vi "main.vi"() -> ()   [LabVIEW 2023] (continued)
1FFFFFFF   00000004    8        00\t00\tFF\tFF\tFF\tFF\tFF\tFF\r\n      3246  18F121F0   00000004    8        09\t33\t00\t00\tFF\tFF\tB0\t01\r\n      3245  18F106A7   00000004    8        00\tF7\tFF\tFF\tFF\tFF\tFF\tB1\r\n      3245  0CF104A7   00000004    8        F0\t60\t22\tFC\tFF\tFF\tFF\t58\r\n      3244  0CF103A7   00000004    8        17\t1F\t08\t60\tB1\t1F\t08\t58\r\n      3244  0CF102A7   00000004    8        30\t75\tE0\t2E\t80\tFF\tFF\tFD\r\n      3243  0C3C4D4A   00000004    8        BE\tFF\tFF\t7F\t18\tFF\tFF\t58\r\n      3272  1FFFFFFF   00000004    8        00\t00\tFF\tFF\tFF\tFF\tFF\tFF\r\n      3263  0CF102A7   00000004    8        30\t75\tE0\t2E\t80\tFF\tFF\tFD\r\n      3263  0CF101A7   00000004    8        68\t00\t97\tCC\t00\t19\t39\tBD\r\n      3262  1FFFFFFF   00000004    8        00\t00\tFF\tFF\tFF\tFF\tFF\tFF\r\n      3252  1FFFFFFF   00000004    8        00\t00\tFF\tFF\tFF\tFF\tFF\tFF\r\n      3247  1FFFFFFF   00000004    8        00\t00\tFF\tFF\tFF\tFF\tFF\tFF\r\n      3246  18F121F0   00000004    8        09\t33\t00\t00\tFF\tFF\tB0\t01\r\n      3245  18F106A7   00000004    8        00\tF7\tFF\tFF\tFF\tFF\tFF\tB1\r\n      3245  0CF104A7   00000004    8        F0\t60\t22\tFC\tFF\tFF\tFF\t58\r\n      3244  0CF103A7   00000004    8        17\t1F\t08\t60\tB1\t1F\t08\t58\r\n      3244  0CF102A7   00000004    8        30\t75\tE0\t2E\t80\tFF\tFF\tFD\r\n      3282  1FFFFFFF   00000004    8        00\t00\tFF\tFF\tFF\tFF\tFF\tFF\r\n      3272  1FFFFFFF   00000004    8        00\t00\tFF\tFF\tFF\tFF\tFF\tFF\r\n      3263  0CF102A7   00000004    8        30\t75\tE0\t2E\t80\tFF\tFF\tFD\r\n      3263  0CF101A7   00000004    8        68\t00\t97\tCC\t00\t19\t39\tBD\r\n      3262  1FFFFFFF   00000004    8        00\t00\tFF\tFF\tFF\tFF\tFF\tFF\r\n      3252  1FFFFFFF   00000004    8        00\t00\tFF\tFF\tFF\tFF\tFF\tFF\r\n      3247  1FFFFFFF   00000004    8        00\t00\tFF\tFF\tFF\tFF\tFF\tFF\r\n      3246  18F121F0   00000004    8        09\t33\t00\t00\tFF\tFF\tB0\t01\r\n      3245  18F106A7   00000004    8        00\tF7\tFF\tFF\tFF\tFF\tFF\tB1\r\n      3245  0CF104A7   00000004    8        F0\t60\t22\tFC\tFF\tFF\tFF\t58\r\n      3244  0CF103A7   00000004    8        17\t1F\t08\t60\tB1\t1F\t08\t58\r\n      3283  0CF101A7   00000004    8        68\t00\t97\tCC\t00\t19\t39\tBE\r\n      3282  1FFFFFFF   00000004    8        00\t00\tFF\tFF\tFF\tFF\tFF\tFF\r\n      3272  1FFFFFFF   00000004    8        00\t00\tFF\tFF\tFF\tFF\tFF\tFF\r\n      3263  0CF102A7   00000004    8        30\t75\tE0\t2E\t80\tFF\tFF\tFD\r\n      3263  0CF101A7   00000004    8        68\t00\t97\tCC\t00\t19\t39\tBD\r\n      3262  1FFFFFFF   00000004    8        00\t00\tFF\tFF\tFF\tFF\tFF\tFF\r\n      3252  1FFFFFFF   00000004    8        00\t00\tFF\tFF\tFF\tFF\tFF\tFF\r\n      3247  1FFFFFFF   00000004    8        00\t00\tFF\tFF\tFF\tFF\tFF\tFF\r\n      3246  18F121F0   00000004    8        09\t33\t00\t00\tFF\tFF\tB0\t01\r\n      3245  18F106A7   00000004    8        00\tF7\tFF\tFF\tFF\tFF\tFF\tB1\r\n      3245  0CF104A7   00000004    8        F0\t60\t22\tFC\tFF\tFF\tFF\t58\r\n      3283  0CF102A7   00000004    8        30\t75\tE0\t2E\t80\tFF\tFF\tFD\r\n      3283  0CF101A7   00000004    8        68\t00\t97\tCC\t00\t19\t39\tBE\r\n      3282  1FFFFFFF   00000004    8        00\t00\tFF\tFF\tFF\tFF\tFF\tFF\r\n      3272  1FFFFFFF   00000004    8        00\t00\tFF\tFF\tFF\tFF\tFF\tFF\r\n      3263  0CF102A7   00000004    8        30\t75\tE0\t2E\t80\tFF\tFF\tFD\r\n      3263  0CF101A7   00000004    8        68\t00\t97\tCC\t00\t19\t39\tBD\r\n      3262  1FFFFFFF   00000004    8        00\t00\tFF\tFF\tFF\tFF\tFF\tFF\r\n      3252  1FFFFFFF   00000004    8        00\t00\tFF\tFF\tFF\tFF\tFF\tFF\r\n      3247  1FFFFFFF   00000004    8        00\t00\tFF\tFF\tFF\tFF\tFF\tFF\r\n      3246  18F121F0   00000004    8        09\t33\t00\t00\tFF\tFF\tB0\t01\r\n      3245  18F106A7   00000004    8        00\tF7\tFF\tFF\tFF\tFF\tFF\tB1\r\n      3292  1FFFFFFF   00000004    8        00\t00\tFF\tFF\tFF\tFF\tFF\tFF\r\n      3283  0CF102A7   00000004    8        30\t75\tE0\t2E\t80\tFF\tFF\tFD\r\n      3283  0CF101A7   00000004    8        68\t00\t97\tCC\t00\t19\t39\tBE\r\n      3282  1FFFFFFF   00000004    8        00\t00\tFF\tFF\tFF\tFF\tFF\tFF\r\n      3272  1FFFFFFF   00000004    8        00\t00\tFF\tFF\tFF\tFF\tFF\tFF\r\n      3263  0CF102A7   00000004    8        30\t75\tE0\t2E\t80\tFF\tFF\tFD\r\n      3263  0CF101A7   00000004    8        68\t00\t97\tCC\t00\t19\t39\tBD\r\n      3262  1FFFFFFF   00000004    8        00\t00\tFF\tFF\tFF\tFF\tFF\tFF\r\n      3252  1FFFFFFF   00000004    8        00\t00\tFF\tFF\tFF\tFF\tFF\tFF\r\n      3247  1FFFFFFF   00000004    8        00\t00\tFF\tFF\tFF\tFF\tFF\tFF\r\n      3246  18F121F0   00000004    8        09\t33\t00\t00\tFF\tFF\tB0\t01\r\n      3293  18F106A7   00000004    8        00\tF7\tFF\tFF\tFF\tFF\tFF\tB2\r\n      3292  1FFFFFFF   00000004    8        00\t00\tFF\tFF\tFF\tFF\tFF\tFF\r\n      3283  0CF102A7   00000004    8        30\t75\tE0\t2E\t80\tFF\tFF\tFD\r\n      3283  0CF101A7   00000004    8        68\t00\t97\tCC\t00\t19\t39\tBE\r\n      3282  1FFFFFFF   00000004    8        00\t00\tFF\tFF\tFF\tFF\tFF\tFF\r\n      3272  1FFFFFFF   00000004    8        00\t00\tFF\tFF\tFF\tFF\tFF\tFF\r\n      3263  0CF102A7   00000004    8        30\t75\tE0\t2E\t80\tFF\tFF\tFD\r\n      3263  0CF101A7   00000004    8        68\t00\t97\tCC\t00\t19\t39\tBD\r\n      3262  1FFFFFFF   00000004    8        00\t00\tFF\tFF\tFF\tFF\tFF\tFF\r\n      3252  1FFFFFFF   00000004    8        00\t00\tFF\tFF\tFF\tFF\tFF\tFF\r\n      3247  1FFFFFFF   00000004    8        00\t00\tFF\tFF\tFF\tFF\tFF\tFF\r\n      3302  1FFFFFFF   00000004    8        00\t00\tFF\tFF\tFF\tFF\tFF\tFF\r\n      3293  18F106A7   00000004    8        00\tF7\tFF\tFF\tFF\tFF\tFF\tB2\r\n      3292  1FFFFFFF   00000004    8        00\t00\tFF\tFF\tFF\tFF\tFF\tFF\r\n      3283  0CF102A7   00000004    8        30\t75\tE0\t2E\t80\tFF\tFF\tFD\r\n      3283  0CF101A7   00000004    8        68\t00\t97\tCC\t00\t19\t39\tBE\r\n      3282  1FFFFFFF   00000004    8        00\t00\tFF\tFF\tFF\tFF\tFF\tFF\r\n      3272  1FFFFFFF   00000004    8        00\t00\tFF\tFF\tFF\tFF\tFF\tFF\r\n      3263  0CF102A7   00000004    8        30\t75\tE0\t2E\t80\tFF\tFF\tFD\r\n      3263  0CF101A7   00000004    8        68\t00\t97\tCC\t00\t19\t39\tBD\r\n      3262  1FFFFFFF   00000004    8        00\t00\tFF\tFF\tFF\tFF\tFF\tFF\r\n      3252  1FFFFFFF   00000004    8        00\t00\tFF\tFF\tFF\tFF\tFF\tFF\r\n      3303  0CF101A7   00000004    8        68\t00\t97\tCC\t00\t19\t39\tBF\r\n      3302  1FFFFFFF   00000004    8        00\t00\tFF\tFF\tFF\tFF\tFF\tFF\r\n      3293  18F106A7   00000004    8        00\tF7\tFF\tFF\tFF\tFF\tFF\tB2\r\n      3292  1FFFFFFF   00000004    8        00\t00\tFF\tFF\tFF\tFF\tFF\tFF\r\n      3283  0CF102A7   00000004    8        30\t75\tE0\t2E\t80\tFF\tFF\tFD\r\n      3283  0CF101A7   00000004    8        68\t00\t97\tCC\t00\t19\t39\tBE\r\n      3282  1FFFFFFF   00000004    8        00\t00\tFF\tFF\tFF\tFF\tFF\tFF\r\n      3272  1FFFFFFF   00000004    8        00\t00\tFF\tFF\tFF\tFF\tFF\tFF\r\n      3263  0CF102A7   00000004    8        30\t75\tE0\t2E\t80\tFF\tFF\tFD\r\n      3263  0CF101A7   00000004    8        68\t00\t97\tCC\t00\t19\t39\tBD\r\n      3262  1FFFFFFF   00000004    8        00\t00\tFF\tFF\tFF\tFF\tFF\tFF\r\n      3303  0CF102A7   00000004    8        30\t75\tE0\t2E\t80\tFF\tFF\tFD\r\n      3303  0CF101A7   00000004    8        68\t00\t97\tCC\t00\t19\t39\tBF\r\n      3302  1FFFFFFF   00000004    8        00\t00\tFF\tFF\tFF\tFF\tFF\tFF\r\n      3293  18F106A7   00000004    8        00\tF7\tFF\tFF\tFF\tFF\tFF\tB2\r\n      3292  1FFFFFFF   00000004    8        00\t00\tFF\tFF\tFF\tFF\tFF\tFF\r\n      3283  0CF102A7   00000004    8        30\t75\tE0\t2E\t80\tFF\tFF\tFD\r\n      3283  0CF101A7   00000004    8        68\t00\t97\tCC\t00\t19\t39\tBE\r\n      3282  1FFFFFFF   00000004    8        00\t00\tFF\tFF\tFF\tFF\tFF\tFF\r\n      3272  1FFFFFFF   00000004    8        00\t00\tFF\tFF\tFF\tFF\tFF\tFF\r\n      3263  0CF102A7   00000004    8        30\t75\tE0\t2E\t80\tFF\tFF\tFD\r\n      3263  0CF101A7   00000004    8        68\t00\t97\tCC\t00\t19\t39\tBD\r\n      3312  1FFFFFFF   00000004    8        00\t20\tFF\tFF\tFF\tFF\tFF\tFF\r\n      3303  0CF102A7   00000004    8        30\t75\tE0\t2E\t80\tFF\tFF\tFD\r\n      3303  0CF101A7   00000004    8        68\t00\t97\tCC\t00\t19\t39\tBF\r\n      3302  1FFFFFFF   00000004    8        00\t00\tFF\tFF\tFF\tFF\tFF\tFF\r\n      3293  18F106A7   00000004    8        00\tF7\tFF\tFF\tFF\tFF\tFF\tB2\r\n      3292  1FFFFFFF   00000004    8        00\t00\tFF\tFF\tFF\tFF\tFF\tFF\r\n      3283  0CF102A7   00000004    8        30\t75\tE0\t2E\t80\tFF\tFF\tFD\r\n      3283  0CF101A7   00000004    8        68\t00\t97\tCC\t00\t19\t39\tBE\r\n      3282  1FFFFFFF   00000004    8        00\t00\tFF\tFF\tFF\tFF\tFF\tFF\r\n      3272  1FFFFFFF   00000004    8        00\t00\tFF\tFF\tFF\tFF\tFF\tFF\r\n      3263  0CF102A7   00000004    8        30\t75\tE0\t2E\t80\tFF\tFF\tFD\r\n      3322  1FFFFFFF   00000004    8        00\t00\tFF\tFF\tFF\tFF\tFF\tFF\r\n      3312  1FFFFFFF   00000004    8        00\t20\tFF\tFF\tFF\tFF\tFF\tFF\r\n      3303  0CF102A7   00000004    8        30\t75\tE0\t2E\t80\tFF\tFF\tFD\r\n      3303  0CF101A7   00000004    8        68\t00\t97\tCC\t00\t19\t39\tBF\r\n      3302  1FFFFFFF   00000004    8        00\t00\tFF\tFF\tFF\tFF\tFF\tFF\r\n      3293  18F106A7   00000004    8        00\tF7\tFF\tFF\tFF\tFF\tFF\tB2\r\n      3292  1FFFFFFF   00000004    8        00\t00\tFF\tFF\tFF\tFF\tFF\tFF\r\n      3283  0CF102A7   00000004    8        30\t75\tE0\t2E\t80\tFF\tFF\tFD\r\n      3283  0CF101A7   00000004    8        68\t00\t97\tCC\t00\t19\t39\tBE\r\n      3282  1FFFFFFF   00000004    8        00\t00\tFF\tFF\tFF\tFF\tFF\tFF\r\n      3272  1FFFFFFF   00000004    8        00\t00\tFF\tFF\tFF\tFF\tFF\tFF\r\n      3323  0CF101A7   00000004    8        68\t00\t97\tCC\t00\t19\t39\tC0\r\n      3322  1FFFFFFF   00000004    8        00\t00\tFF\tFF\tFF\tFF\tFF\tFF\r\n      3312  1FFFFFFF   00000004    8        00\t20\tFF\tFF\tFF\tFF\tFF\tFF\r\n      3303  0CF102A7   00000004    8        30\t75\tE0\t2E\t80\tFF\tFF\tFD\r\n      3303  0CF101A7   00000004    8        68\t00\t97\tCC\t00\t19\t39\tBF\r\n      3302  1FFFFFFF   00000004    8        00\t00\tFF\tFF\tFF\tFF\tFF\tFF\r\n      3293  18F106A7   00000004    8        00\tF7\tFF\tFF\tFF\tFF\tFF\tB2\r\n      3292  1FFFFFFF   00000004    8        00\t00\tFF\tFF\tFF\tFF\tFF\tFF\r\n      3283  0CF102A7   00000004    8        30\t75\tE0\t2E\t80\tFF\tFF\tFD\r\n      3283  0CF101A7   00000004    8        68\t00\t97\tCC\t00\t19\t39\tBE\r\n      3282  1FFFFFFF   00000004    8        00\t00\tFF\tFF\tFF\tFF\tFF\tFF\r\n      3323  0CF102A7   00000004    8        30\t75\tE0\t2E\t80\tFF\tFF\tFD\r\n      3323  0CF101A7   00000004    8        68\t00\t97\tCC\t00\t19\t39\tC0\r\n      3322  1FFFFFFF   00000004    8        00\t00\tFF\tFF\tFF\tFF\tFF\tFF\r\n      3312  1FFFFFFF   00000004    8        00\t20\tFF\tFF\tFF\tFF\tFF\tFF\r\n      3303  0CF102A7   00000004    8        30\t75\tE0\t2E\t80\tFF\tFF\tFD\r\n      3303  0CF101A7   00000004    8        68\t00\t97\tCC\t00\t19\t39\tBF\r\n      3302  1FFFFFFF   00000004    8        00\t00\tFF\tFF\tFF\tFF\tFF\tFF\r\n      3293  18F106A7   00000004    8        00\tF7\tFF\tFF\tFF\tFF\tFF\tB2\r\n      3292  1FFFFFFF   00000004    8        00\t00\tFF\tFF\tFF\tFF\tFF\tFF\r\n      3283  0CF102A7   00000004    8        30\t75\tE0\t2E\t80\tFF\tFF\tFD\r\n      3283  0CF101A7   00000004    8        68\t00\t97\tCC\t00\t19\t39\tBE\r\n      3332  1FFFFFFF   00000004    8        00\t00\tFF\tFF\tFF\tFF\tFF\tFF\r\n      3323  0CF102A7   00000004    8        30\t75\tE0\t2E\t80\tFF\tFF\tFD\r\n      3323  0CF101A7   00000004    8        68\t00\t97\tCC\t00\t19\t39\tC0\r\n      3322  1FFFFFFF   00000004    8        00\t00\tFF\tFF\tFF\tFF\tFF\tFF\r\n      3312  1FFFFFFF   00000004    8        00\t20\tFF\tFF\tFF\tFF\tFF\tFF\r\n      3303  0CF102A7   00000004    8        30\t75\tE0\t2E\t80\tFF\tFF\tFD\r\n      3303  0CF101A7   00000004    8        68\t00\t97\tCC\t00\t19\t39\tBF\r\n      3302  1FFFFFFF   00000004    8        00\t00\tFF\tFF\tFF\tFF\tFF\tFF\r\n      3293  18F106A7   00000004    8        00\tF7\tFF\tFF\tFF\tFF\tFF\tB2\r\n      3292  1FFFFFFF   00000004    8        00\t00\tFF\tFF\tFF\tFF\tFF\tFF\r\n      3283  0CF102A7   00000004    8        30\t75\tE0\t2E\t80\tFF\tFF\tFD\r\n      3341  18F11FF0   00000004    8        FF\t3F\t90\t68\t88\t1B\t10\t9C\r\n      3332  1FFFFFFF   00000004    8        00\t00\tFF\tFF\tFF\tFF\tFF\tFF\r\n      3323  0CF102A7   00000004    8        30\t75\tE0\t2E\t80\tFF\tFF\tFD\r\n      3323  0CF101A7   00000004    8        68\t00\t97\tCC\t00\t19\t39\tC0\r\n      3322  1FFFFFFF   00000004    8        00\t00\tFF\tFF\tFF\tFF\tFF\tFF\r\n      3312  1FFFFFFF   00000004    8        00\t20\tFF\tFF\tFF\tFF\tFF\tFF\r\n      3303  0CF102A7   00000004    8        30\t75\tE0\t2E\t80\tFF\tFF\tFD\r\n      3303  0CF101A7   00000004    8        68\t00\t97\tCC\t00\t19\t39\tBF\r\n      3302  1FFFFFFF   00000004    8        00\t00\tFF\tFF\tFF\tFF\tFF\tFF\r\n      3293  18F106A7   00000004    8        00\tF7\tFF\tFF\tFF\tFF\tFF\tB2\r\n      3292  1FFFFFFF   00000004    8        00\t00\tFF\tFF\tFF\tFF\tFF\tFF\r\n      3342  18F120F0   00000004    8        2B\t75\t60\tB1\tB0\t01\tFF\tFF\r\n      3341  18F11FF0   00000004    8        FF\t3F\t90\t68\t88\t1B\t10\t9C\r\n      3332  1FFFFFFF   00000004    8        00\t00\tFF\tFF\tFF\tFF\tFF\tFF\r\n      3323  0CF102A7   00000004    8        30\t75\tE0\t2E\t80\tFF\tFF\tFD\r\n      3323  0CF101A7   00000004    8        68\t00\t97\tCC\t00\t19\t39\tC0\r\n      3322  1FFFFFFF   00000004    8        00\t00\tFF\tFF\tFF\tFF\tFF\tFF\r\n      3312  1FFFFFFF   00000004    8        00\t20\tFF\tFF\tFF\tFF\tFF\tFF\r\n      3303  0CF102A7   00000004    8        30\t75\tE0\t2E\t80\tFF\tFF\tFD\r\n      3303  0CF101A7   00000004    8        68\t00\t97\tCC\t00\t19\t39\tBF\r\n      3302  1FFFFFFF   00000004    8        00\t00\tFF\tFF\tFF\tFF\tFF\tFF\r\n      3293  18F106A7   00000004    8        00\tF7\tFF\tFF\tFF\tFF\tFF\tB2\r\n      3343  0CF101A7   00000004    8        68\t00\t97\tCC\t00\t19\t39\tC1\r\n      3342  18F120F0   00000004    8        2B\t75\t60\tB1\tB0\t01\tFF\tFF\r\n      3341  18F11FF0   00000004    8        FF\t3F\t90\t68\t88\t1B\t10\t9C\r\n      3332  1FFFFFFF   00000004    8        00\t00\tFF\tFF\tFF\tFF\tFF\tFF\r\n      3323  0CF102A7   00000004    8        30\t75\tE0\t2E\t80\tFF\tFF\tFD\r\n      3323  0CF101A7   00000004    8        68\t00\t97\tCC\t00\t19\t39\tC0\r\n      3322  1FFFFFFF   00000004    8        00\t00\tFF\tFF\tFF\tFF\tFF\tFF\r\n      3312  1FFFFFFF   00000004    8        00\t20\tFF\tFF\tFF\tFF\tFF\tFF\r\n      3303  0CF102A7   00000004    8        30\t75\tE0\t2E\t80\tFF\tFF\tFD\r\n      3303  0CF101A7   00000004    8        68\t00\t97\tCC\t00\t19\t39\tBF\r\n      3302  1FFFFFFF   00000004    8        00\t00\tFF\tFF\tFF\tFF\tFF\tFF\r\n      3343  0C3C4D4A   00000004    8        BE\tFF\tFF\t7F\t18\tFF\tFF\t59\r\n      3343  0CF101A7   00000004    8        68\t00\t97\tCC\t00\t19\t39\tC1\r\n      3342  18F120F0   00000004    8        2B\t75\t60\tB1\tB0\t01\tFF\tFF\r\n      3341  18F11FF0   00000004    8        FF\t3F\t90\t68\t88\t1B\t10\t9C\r\n      3332  1FFFFFFF   00000004    8        00\t00\tFF\tFF\tFF\tFF\tFF\tFF\r\n      3323  0CF102A7   00000004    8        30\t75\tE0\t2E\t80\tFF\tFF\tFD\r\n      3323  0CF101A7   00000004    8        68\t00\t97\tCC\t00\t19\t39\tC0\r\n      3322  1FFFFFFF   00000004    8        00\t00\tFF\tFF\tFF\tFF\tFF\tFF\r\n      3312  1FFFFFFF   00000004    8        00\t20\tFF\tFF\tFF\tFF\tFF\tFF\r\n      3303  0CF102A7   00000004    8        30\t75\tE0\t2E\t80\tFF\tFF\tFD\r\n      3303  0CF101A7   00000004    8        68\t00\t97\tCC\t00\t19\t39\tBF\r\n      3344  0CF102A7   00000004    8        30\t75\tE0\t2E\t80\tFF\tFF\tFD\r\n      3343  0C3C4D4A   00000004    8        BE\tFF\tFF\t7F\t18\tFF\tFF\t59\r\n      3343  0CF101A7   00000004    8        68\t00\t97\tCC\t00\t19\t39\tC1\r\n      3342  18F120F0   00000004    8        2B\t75\t60\tB1\tB0\t01\tFF\tFF\r\n      3341  18F11FF0   00000004    8        FF\t3F\t90\t68\t88\t1B\t10\t9C\r\n      3332  1FFFFFFF   00000004    8        00\t00\tFF\tFF\tFF\tFF\tFF\tFF\r\n      3323  0CF102A7   00000004    8        30\t75\tE0\t2E\t80\tFF\tFF\tFD\r\n      3323  0CF101A7   00000004    8        68\t00\t97\tCC\t00\t19\t39\tC0\r\n      3322  1FFFFFFF   00000004    8        00\t00\tFF\tFF\tFF\tFF\tFF\tFF\r\n      3312  1FFFFFFF   00000004    8        00\t20\tFF\tFF\tFF\tFF\tFF\tFF\r\n      3303  0CF102A7   00000004    8        30\t75\tE0\t2E\t80\tFF\tFF\tFD\r\n      3344  0CF103A7   00000004    8        17\t1F\t08\t60\tB1\t1F\t08\t59\r\n      3344  0CF102A7   00000004    8        30\t75\tE0\t2E\t80\tFF\tFF\tFD\r\n      3343  0C3C4D4A   00000004    8        BE\tFF\tFF\t7F\t18\tFF\tFF\t59\r\n      3343  0CF101A7   00000004    8        68\t00\t97\tCC\t00\t19\t39\tC1\r\n      3342  18F120F0   00000004    8        2B\t75\t60\tB1\tB0\t01\tFF\tFF\r\n      3341  18F11FF0   00000004    8        FF\t3F\t90\t68\t88\t1B\t10\t9C\r\n      3332  1FFFFFFF   00000004    8        00\t00\tFF\tFF\tFF\tFF\tFF\tFF\r\n      3323  0CF102A7   00000004    8        30\t75\tE0\t2E\t80\tFF\tFF\tFD\r\n      3323  0CF101A7   00000004    8        68\t00\t97\tCC\t00\t19\t39\tC0\r\n      3322  1FFFFFFF   00000004    8        00\t00\tFF\tFF\tFF\tFF\tFF\tFF\r\n      3312  1FFFFFFF   00000004    8        00\t20\tFF\tFF\tFF\tFF\tFF\tFF\r\n      3345  0CF104A7   00000004    8        F0\t60\t22\tFC\tFF\tFF\tFF\t59\r\n      3344  0CF103A7   00000004    8        17\t1F\t08\t60\tB1\t1F\t08\t59\r\n      3344  0CF102A7   00000004    8        30\t75\tE0\t2E\t80\tFF\tFF\tFD\r\n      3343  0C3C4D4A   00000004    8        BE\tFF\tFF\t7F\t18\tFF\tFF\t59\r\n      3343  0CF101A7   00000004    8        68\t00\t97\tCC\t00\t19\t39\tC1\r\n      3342  18F120F0   00000004    8        2B\t75\t60\tB1\tB0\t01\tFF\tFF\r\n      3341  18F11FF0   00000004    8        FF\t3F\t90\t68\t88\t1B\t10\t9C\r\n      3332  1FFFFFFF   00000004    8        00\t00\tFF\tFF\tFF\tFF\tFF\tFF\r\n      3323  0CF102A7   00000004    8        30\t75\tE0\t2E\t80\tFF\tFF\tFD\r\n      3323  0CF101A7   00000004    8        68\t00\t97\tCC\t00\t19\t39\tC0\r\n      3322  1FFFFFFF   00000004    8        00\t00\tFF\tFF\tFF\tFF\tFF\tFF\r\n      3345  18F106A7   00000004    8        00\tF7\tFF\tFF\tFF\tFF\tFF\tB3\r\n      3345  0CF104A7   00000004    8        F0\t60\t22\tFC\tFF\tFF\tFF\t59\r\n      3344  0CF103A7   00000004    8        17\t1F\t08\t60\tB1\t1F\t08\t59\r\n      3344  0CF102A7   00000004    8        30\t75\tE0\t2E\t80\tFF\tFF\tFD\r\n      3343  0C3C4D4A   00000004    8        BE\tFF\tFF\t7F\t18\tFF\tFF\t59\r\n      3343  0CF101A7   00000004    8        68\t00\t97\tCC\t00\t19\t39\tC1\r\n      3342  18F120F0   00000004    8        2B\t75\t60\tB1\tB0\t01\tFF\tFF\r\n      3341  18F11FF0   00000004    8        FF\t3F\t90\t68\t88\t1B\t10\t9C\r\n      3332  1FFFFFFF   00000004    8        00\t00\tFF\tFF\tFF\tFF\tFF\tFF\r\n      3323  0CF102A7   00000004    8        30\t75\tE0\t2E\t80\tFF\tFF\tFD\r\n      3323  0CF101A7   00000004    8        68\t00\t97\tCC\t00\t19\t39\tC0\r\n      3346  18F121F0   00000004    8        09\t33\t00\t00\tFF\tFF\tB0\t01\r\n      3345  18F106A7   00000004    8        00\tF7\tFF\tFF\tFF\tFF\tFF\tB3\r\n      3345  0CF104A7   00000004    8        F0\t60\t22\tFC\tFF\tFF\tFF\t59\r\n      3344  0CF103A7   00000004    8        17\t1F\t08\t60\tB1\t1F\t08\t59\r\n      3344  0CF102A7   00000004    8        30\t75\tE0\t2E\t80\tFF\tFF\tFD\r\n      3343  0C3C4D4A   00000004    8        BE\tFF\tFF\t7F\t18\tFF\tFF\t59\r\n      3343  0CF101A7   00000004    8        68\t00\t97\tCC\t00\t19\t39\tC1\r\n      3342  18F120F0   00000004    8        2B\t75\t60\tB1\tB0\t01\tFF\tFF\r\n      3341  18F11FF0   00000004    8        FF\t3F\t90\t68\t88\t1B\t10\t9C\r\n      3332  1FFFFFFF   00000004    8        00\t00\tFF\tFF\tFF\tFF\tFF\tFF\r\n      3323  0CF102A7   00000004    8        30\t75\tE0\t2E\t80\tFF\tFF\tFD\r\n      3347  1FFFFFFF   00000004    8        00\t00\tFF\tFF\tFF\tFF\tFF\tFF\r\n      3346  18F121F0   00000004    8        09\t33\t00\t00\tFF\tFF\tB0\t01\r\n      3345  18F106A7   00000004    8        00\tF7\tFF\tFF\tFF\tFF\tFF\tB3\r\n      3345  0CF104A7   00000004    8        F0\t60\t22\tFC\tFF\tFF\tFF\t59\r\n      3344  0CF103A7   00000004    8        17\t1F\t08\t60\tB1\t1F\t08\t59\r\n      3344  0CF102A7   00000004    8        30\t75\tE0\t2E\t80\tFF\tFF\tFD\r\n      3343  0C3C4D4A   00000004    8        BE\tFF\tFF\t7F\t18\tFF\tFF\t59\r\n      3343  0CF101A7   00000004    8        68\t00\t97\tCC\t00\t19\t39\tC1\r\n      3342  18F120F0   00000004    8        2B\t75\t60\tB1\tB0\t01\tFF\tFF\r\n      3341  18F11FF0   00000004    8        FF\t3F\t90\t68\t88\t1B\t10\t9C\r\n      3332  1FFFFFFF   00000004    8        00\t00\tFF\tFF\tFF\tFF\tFF\tFF\r\n      3352  1FFFFFFF   00000004    8        00\t00\tFF\tFF\tFF\tFF\tFF\tFF\r\n      3347  1FFFFFFF   00000004    8        00\t00\tFF\tFF\tFF\tFF\tFF\tFF\r\n      3346  18F121F0   00000004    8        09\t33\t00\t00\tFF\tFF\tB0\t01\r\n      3345  18F106A7   00000004    8        00\tF7\tFF\tFF\tFF\tFF\tFF\tB3\r\n      3345  0CF104A7   00000004    8        F0\t60\t22\tFC\tFF\tFF\tFF\t59\r\n      3344  0CF103A7   00000004    8        17\t1F\t08\t60\tB1\t1F\t08\t59\r\n      3344  0CF102A7   00000004    8        30\t75\tE0\t2E\t80\tFF\tFF\tFD\r\n      3343  0C3C4D4A   00000004    8        BE\tFF\tFF\t7F\t18\tFF\tFF\t59\r\n      3343  0CF101A7   00000004    8        68\t00\t97\tCC\t00\t19\t39\tC1\r\n      3342  18F120F0   00000004    8        2B\t75\t60\tB1\tB0\t01\tFF\tFF\r\n      3341  18F11FF0   00000004    8        FF\t3F\t90\t68\t88\t1B\t10\t9C\r\n      3362  1FFFFFFF   00000004    8        00\t00\tFF\tFF\tFF\tFF\tFF\tFF\r\n      3352  1FFFFFFF   00000004    8        00\t00\tFF\tFF\tFF\tFF\tFF\tFF\r\n      3347  1FFFFFFF   00000004    8        00\t00\tFF\tFF\tFF\tFF\tFF\tFF\r\n      3346  18F121F0   00000004    8        09\t33\t00\t00\tFF\tFF\tB0\t01\r\n      3345  18F106A7   00000004    8        00\tF7\tFF\tFF\tFF\tFF\tFF\tB3\r\n      3345  0CF104A7   00000004    8        F0\t60\t22\tFC\tFF\tFF\tFF\t59\r\n      3344  0CF103A7   00000004    8        17\t1F\t08\t60\tB1\t1F\t08\t59\r\n      3344  0CF102A7   00000004    8        30\t75\tE0\t2E\t80\tFF\tFF\tFD\r\n      3343  0C3C4D4A   00000004    8        BE\tFF\tFF\t7F\t18\tFF\tFF\t59\r\n      3343  0CF101A7   00000004    8        68\t00\t97\tCC\t00\t19\t39\tC1\r\n      3342  18F120F0   00000004    8        2B\t75\t60\tB1\tB0\t01\tFF\tFF\r\n      3363  0CF101A7   00000004    8        68\t00\t97\tCC\t00\t19\t39\tC2\r\n      3362  1FFFFFFF   00000004    8        00\t00\tFF\tFF\tFF\tFF\tFF\tFF\r\n      3352  1FFFFFFF   00000004    8        00\t00\tFF\tFF\tFF\tFF\tFF\tFF\r\n      3347  1FFFFFFF   00000004    8        00\t00\tFF\tFF\tFF\tFF\tFF\tFF\r\n      3346  18F121F0   00000004    8        09\t33\t00\t00\tFF\tFF\tB0\t01\r\n      3345  18F106A7   00000004    8        00\tF7\tFF\tFF\tFF\tFF\tFF\tB3\r\n      3345  0CF104A7   00000004    8        F0\t60\t22\tFC\tFF\tFF\tFF\t59\r\n      3344  0CF103A7   00000004    8        17\t1F\t08\t60\tB1\t1F\t08\t59\r\n      3344  0CF102A7   00000004    8        30\t75\tE0\t2E\t80\tFF\tFF\tFD\r\n      3343  0C3C4D4A   00000004    8        BE\tFF\tFF\t7F\t18\tFF\tFF\t59\r\n      3343  0CF101A7   00000004    8        68\t00\t97\tCC\t00\t19\t39\tC1\r\n      3363  0CF102A7   00000004    8        30\t75\tE0\t2E\t80\tFF\tFF\tFD\r\n      3363  0CF101A7   00000004    8        68\t00\t97\tCC\t00\t19\t39\tC2\r\n      3362  1FFFFFFF   00000004    8        00\t00\tFF\tFF\tFF\tFF\tFF\tFF\r\n      3352  1FFFFFFF   00000004    8        00\t00\tFF\tFF\tFF\tFF\tFF\tFF\r\n      3347  1FFFFFFF   00000004    8        00\t00\tFF\tFF\tFF\tFF\tFF\tFF\r\n      3346  18F121F0   00000004    8        09\t33\t00\t00\tFF\tFF\tB0\t01\r\n      3345  18F106A7   00000004    8        00\tF7\tFF\tFF\tFF\tFF\tFF\tB3\r\n      3345  0CF104A7   00000004    8        F0\t60\t22\tFC\tFF\tFF\tFF\t59\r\n      3344  0CF103A7   00000004    8        17\t1F\t08\t60\tB1\t1F\t08\t59\r\n      3344  0CF102A7   00000004    8        30\t75\tE0\t2E\t80\tFF\tFF\tFD\r\n      3343  0C3C4D4A   00000004    8        BE\tFF\tFF\t7F\t18\tFF\tFF\t59\r\n      3372  1FFFFFFF   00000004    8        00\t20\tFF\tFF\tFF\tFF\tFF\tFF\r\n      3363  0CF102A7   00000004    8        30\t75\tE0\t2E\t80\tFF\tFF\tFD\r\n      3363  0CF101A7   00000004    8        68\t00\t97\tCC\t00\t19\t39\tC2\r\n      3362  1FFFFFFF   00000004    8        00\t00\tFF\tFF\tFF\tFF\tFF\tFF\r\n      3352  1FFFFFFF   00000004    8        00\t00\tFF\tFF\tFF\tFF\tFF\tFF\r\n      3347  1FFFFFFF   00000004    8        00\t00\tFF\tFF\tFF\tFF\tFF\tFF\r\n      3346  18F121F0   00000004    8        09\t33\t00\t00\tFF\tFF\tB0\t01\r\n      3345  18F106A7   00000004    8        00\tF7\tFF\tFF\tFF\tFF\tFF\tB3\r\n      3345  0CF104A7   00000004    8        F0\t60\t22\tFC\tFF\tFF\tFF\t59\r\n      3344  0CF103A7   00000004    8        17\t1F\t08\t60\tB1\t1F\t08\t59\r\n      3344  0CF102A7   00000004    8        30\t75\tE0\t2E\t80\tFF\tFF\tFD\r\n      3382  1FFFFFFF   00000004    8        00\t00\tFF\tFF\tFF\tFF\tFF\tFF\r\n      3372  1FFFFFFF   00000004    8        00\t20\tFF\tFF\tFF\tFF\tFF\tFF\r\n      3363  0CF102A7   00000004    8        30\t75\tE0\t2E\t80\tFF\tFF\tFD\r\n      3363  0CF101A7   00000004    8        68\t00\t97\tCC\t00\t19\t39\tC2\r\n      3362  1FFFFFFF   00000004    8        00\t00\tFF\tFF\tFF\tFF\tFF\tFF\r\n      3352  1FFFFFFF   00000004    8        00\t00\tFF\tFF\tFF\tFF\tFF\tFF\r\n      3347  1FFFFFFF   00000004    8        00\t00\tFF\tFF\tFF\tFF\tFF\tFF\r\n      3346  18F121F0   00000004    8        09\t33\t00\t00\tFF\tFF\tB0\t01\r\n      3345  18F106A7   00000004    8        00\tF7\tFF\tFF\tFF\tFF\tFF\tB3\r\n      3345  0CF104A7   00000004    8        F0\t60\t22\tFC\tFF\tFF\tFF\t59\r\n      3344  0CF103A7   00000004    8        17\t1F\t08\t60\tB1\t1F\t08\t59\r\n      3383  0CF101A7   00000004    8        68\t00\t97\tCC\t00\t19\t39\tC3\r\n      3382  1FFFFFFF   00000004    8        00\t00\tFF\tFF\tFF\tFF\tFF\tFF\r\n      3372  1FFFFFFF   00000004    8        00\t20\tFF\tFF\tFF\tFF\tFF\tFF\r\n      3363  0CF102A7   00000004    8        30\t75\tE0\t2E\t80\tFF\tFF\tFD\r\n      3363  0CF101A7   00000004    8        68\t00\t97\tCC\t00\t19\t39\tC2\r\n      3362  1FFFFFFF   00000004    8        00\t00\tFF\tFF\tFF\tFF\tFF\tFF\r\n      3352  1FFFFFFF   00000004    8        00\t00\tFF\tFF\tFF\tFF\tFF\tFF\r\n      3347  1FFFFFFF   00000004    8        00\t00\tFF\tFF\tFF\tFF\tFF\tFF\r\n      3346  18F121F0   00000004    8        09\t33\t00\t00\tFF\tFF\tB0\t01\r\n      3345  18F106A7   00000004    8        00\tF7\tFF\tFF\tFF\tFF\tFF\tB3\r\n      3345  0CF104A7   00000004    8        F0\t60\t22\tFC\tFF\tFF\tFF\t59\r\n      3383  0CF102A7   00000004    8        30\t75\tE0\t2E\t80\tFF\tFF\tFD\r\n      3383  0CF101A7   00000004    8        68\t00\t97\tCC\t00\t19\t39\tC3\r\n      3382  1FFFFFFF   00000004    8        00\t00\tFF\tFF\tFF\tFF\tFF\tFF\r\n      3372  1FFFFFFF   00000004    8        00\t20\tFF\tFF\tFF\tFF\tFF\tFF\r\n      3363  0CF102A7   00000004    8        30\t75\tE0\t2E\t80\tFF\tFF\tFD\r\n      3363  0CF101A7   00000004    8        68\t00\t97\tCC\t00\t19\t39\tC2\r\n      3362  1FFFFFFF   00000004    8        00\t00\tFF\tFF\tFF\tFF\tFF\tFF\r\n      3352  1FFFFFFF   00000004    8        00\t00\tFF\tFF\tFF\tFF\tFF\tFF\r\n      3347  1FFFFFFF   00000004    8        00\t00\tFF\tFF\tFF\tFF\tFF\tFF\r\n      3346  18F121F0   00000004    8        09\t33\t00\t00\tFF\tFF\tB0\t01\r\n      3345  18F106A7   00000004    8        00\tF7\tFF\tFF\tFF\tFF\tFF\tB3\r\n      3392  1FFFFFFF   00000004    8        00\t00\tFF\tFF\tFF\tFF\tFF\tFF\r\n      3383  0CF102A7   00000004    8        30\t75\tE0\t2E\t80\tFF\tFF\tFD\r\n      3383  0CF101A7   00000004    8        68\t00\t97\tCC\t00\t19\t39\tC3\r\n      3382  1FFFFFFF   00000004    8        00\t00\tFF\tFF\tFF\tFF\tFF\tFF\r\n      3372  1FFFFFFF   00000004    8        00\t20\tFF\tFF\tFF\tFF\tFF\tFF\r\n      3363  0CF102A7   00000004    8        30\t75\tE0\t2E\t80\tFF\tFF\tFD\r\n      3363  0CF101A7   00000004    8        68\t00\t97\tCC\t00\t19\t39\tC2\r\n      3362  1FFFFFFF   00000004    8        00\t00\tFF\tFF\tFF\tFF\tFF\tFF\r\n      3352  1FFFFFFF   00000004    8        00\t00\tFF\tFF\tFF\tFF\tFF\tFF\r\n      3347  1FFFFFFF   00000004    8        00\t00\tFF\tFF\tFF\tFF\tFF\tFF\r\n      3346  18F121F0   00000004    8        09\t33\t00\t00\tFF\tFF\tB0\t01\r\n      3393  18F106A7   00000004    8        00\tF7\tFF\tFF\tFF\tFF\tFF\tB4\r\n      3392  1FFFFFFF   00000004    8        00\t00\tFF\tFF\tFF\tFF\tFF\tFF\r\n      3383  0CF102A7   00000004    8        30\t75\tE0\t2E\t80\tFF\tFF\tFD\r\n      3383  0CF101A7   00000004    8        68\t00\t97\tCC\t00\t19\t39\tC3\r\n      3382  1FFFFFFF   00000004    8        00\t00\tFF\tFF\tFF\tFF\tFF\tFF\r\n      3372  1FFFFFFF   00000004    8        00\t20\tFF\tFF\tFF\tFF\tFF\tFF\r\n      3363  0CF102A7   00000004    8        30\t75\tE0\t2E\t80\tFF\tFF\tFD\r\n      3363  0CF101A7   00000004    8        68\t00\t97\tCC\t00\t19\t39\tC2\r\n      3362  1FFFFFFF   00000004    8        00\t00\tFF\tFF\tFF\tFF\tFF\tFF\r\n      3352  1FFFFFFF   00000004    8        00\t00\tFF\tFF\tFF\tFF\tFF\tFF\r\n      3347  1FFFFFFF   00000004    8        00\t00\tFF\tFF\tFF\tFF\tFF\tFF\r\n      3402  1FFFFFFF   00000004    8        00\t00\tFF\tFF\tFF\tFF\tFF\tFF\r\n      3393  18F106A7   00000004    8        00\tF7\tFF\tFF\tFF\tFF\tFF\tB4\r\n      3392  1FFFFFFF   00000004    8        00\t00\tFF\tFF\tFF\tFF\tFF\tFF\r\n      3383  0CF102A7   00000004    8        30\t75\tE0\t2E\t80\tFF\tFF\tFD\r\n      3383  0CF101A7   00000004    8        68\t00\t97\tCC\t00\t19\t39\tC3\r\n      3382  1FFFFFFF   00000004    8        00\t00\tFF\tFF\tFF\tFF\tFF\tFF\r\n      3372  1FFFFFFF   00000004    8        00\t20\tFF\tFF\tFF\tFF\tFF\tFF\r\n      3363  0CF102A7   00000004    8        30\t75\tE0\t2E\t80\tFF\tFF\tFD\r\n      3363  0CF101A7   00000004    8        68\t00\t97\tCC\t00\t19\t39\tC2\r\n      3362  1FFFFFFF   00000004    8        00\t00\tFF\tFF\tFF\tFF\tFF\tFF\r\n      3352  1FFFFFFF   00000004    8        00\t00\tFF\tFF\tFF\tFF\tFF\tFF\r\n      3403  0CF101A7   00000004    8        68\t00\t97\tCC\t00\t19\t39\tC4\r\n      3402  1FFFFFFF   00000004    8        00\t00\tFF\tFF\tFF\tFF\tFF\tFF\r\n      3393  18F106A7   00000004    8        00\tF7\tFF\tFF\tFF\tFF\tFF\tB4\r\n      3392  1FFFFFFF   00000004    8        00\t00\tFF\tFF\tFF\tFF\tFF\tFF\r\n      3383  0CF102A7   00000004    8        30\t75\tE0\t2E\t80\tFF\tFF\tFD\r\n      3383  0CF101A7   00000004    8        68\t00\t97\tCC\t00\t19\t39\tC3\r\n      3382  1FFFFFFF   00000004    8        00\t00\tFF\tFF\tFF\tFF\tFF\tFF\r\n      3372  1FFFFFFF   00000004    8        00\t20\tFF\tFF\tFF\tFF\tFF\tFF\r\n      3363  0CF102A7   00000004    8        30\t75\tE0\t2E\t80\tFF\tFF\tFD\r\n      3363  0CF101A7   00000004    8        68\t00\t97\tCC\t00\t19\t39\tC2\r\n      3362  1FFFFFFF   00000004    8        00\t00\tFF\tFF\tFF\tFF\tFF\tFF\r\n      3403  0CF102A7   00000004    8        30\t75\tE0\t2E\t80\tFF\tFF\tFD\r\n      3403  0CF101A7   00000004    8        68\t00\t97\tCC\t00\t19\t39\tC4\r\n      3402  1FFFFFFF   00000004    8        00\t00\tFF\tFF\tFF\tFF\tFF\tFF\r\n      3393  18F106A7   00000004    8        00\tF7\tFF\tFF\tFF\tFF\tFF\tB4\r\n      3392  1FFFFFFF   00000004    8        00\t00\tFF\tFF\tFF\tFF\tFF\tFF\r\n      3383  0CF102A7   00000004    8        30\t75\tE0\t2E\t80\tFF\tFF\tFD\r\n      3383  0CF101A7   00000004    8        68\t00\t97\tCC\t00\t19\t39\tC3\r\n      3382  1FFFFFFF   00000004    8        00\t00\tFF\tFF\tFF\tFF\tFF\tFF\r\n      3372  1FFFFFFF   00000004    8        00\t20\tFF\tFF\tFF\tFF\tFF\tFF\r\n      3363  0CF102A7   00000004    8        30\t75\tE0\t2E\t80\tFF\tFF\tFD\r\n      3363  0CF101A7   00000004    8        68\t00\t97\tCC\t00\t19\t39\tC2\r\n      3412  1FFFFFFF   00000004    8        00\t00\tFF\tFF\tFF\tFF\tFF\tFF\r\n      3403  0CF102A7   00000004    8        30\t75\tE0\t2E\t80\tFF\tFF\tFD\r\n      3403  0CF101A7   00000004    8        68\t00\t97\tCC\t00\t19\t39\tC4\r\n      3402  1FFFFFFF   00000004    8        00\t00\tFF\tFF\tFF\tFF\tFF\tFF\r\n      3393  18F106A7   00000004    8        00\tF7\tFF\tFF\tFF\tFF\tFF\tB4\r\n      3392  1FFFFFFF   00000004    8        00\t00\tFF\tFF\tFF\tFF\tFF\tFF\r\n      3383  0CF102A7   00000004    8        30\t75\tE0\t2E\t80\tFF\tFF\tFD\r\n      3383  0CF101A7   00000004    8        68\t00\t97\tCC\t00\t19\t39\tC3\r\n      3382  1FFFFFFF   00000004    8        00\t00\tFF\tFF\tFF\tFF\tFF\tFF\r\n      3372  1FFFFFFF   00000004    8        00\t20\tFF\tFF\tFF\tFF\tFF\tFF\r\n      3363  0CF102A7   00000004    8        30\t75\tE0\t2E\t80\tFF\tFF\tFD\r\n      3422  1FFFFFFF   00000004    8        00\t00\tFF\tFF\tFF\tFF\tFF\tFF\r\n      3412  1FFFFFFF   00000004    8        00\t00\tFF\tFF\tFF\tFF\tFF\tFF\r\n      3403  0CF102A7   00000004    8        30\t75\tE0\t2E\t80\tFF\tFF\tFD\r\n      3403  0CF101A7   00000004    8        68\t00\t97\tCC\t00\t19\t39\tC4\r\n      3402  1FFFFFFF   00000004    8        00\t00\tFF\tFF\tFF\tFF\tFF\tFF\r\n      3393  18F106A7   00000004    8        00\tF7\tFF\tFF\tFF\tFF\tFF\tB4\r\n      3392  1FFFFFFF   00000004    8        00\t00\tFF\tFF\tFF\tFF\tFF\tFF\r\n      3383  0CF102A7   00000004    8        30\t75\tE0\t2E\t80\tFF\tFF\tFD\r\n      3383  0CF101A7   00000004    8        68\t00\t97\tCC\t00\t19\t39\tC3\r\n      3382  1FFFFFFF   00000004    8        00\t00\tFF\tFF\tFF\tFF\tFF\tFF\r\n      3372  1FFFFFFF   00000004    8        00\t20\tFF\tFF\tFF\tFF\tFF\tFF\r\n      3423  0CF101A7   00000004    8        68\t00\t97\tCC\t00\t19\t39\tC5\r\n      3422  1FFFFFFF   00000004    8        00\t00\tFF\tFF\tFF\tFF\tFF\tFF\r\n      3412  1FFFFFFF   00000004    8        00\t00\tFF\tFF\tFF\tFF\tFF\tFF\r\n      3403  0CF102A7   00000004    8        30\t75\tE0\t2E\t80\tFF\tFF\tFD\r\n      3403  0CF101A7   00000004    8        68\t00\t97\tCC\t00\t19\t39\tC4\r\n      3402  1FFFFFFF   00000004    8        00\t00\tFF\tFF\tFF\tFF\tFF\tFF\r\n      3393  18F106A7   00000004    8        00\tF7\tFF\tFF\tFF\tFF\tFF\tB4\r\n      3392  1FFFFFFF   00000004    8        00\t00\tFF\tFF\tFF\tFF\tFF\tFF\r\n      3383  0CF102A7   00000004    8        30\t75\tE0\t2E\t80\tFF\tFF\tFD\r\n      3383  0CF101A7   00000004    8        68\t00\t97\tCC\t00\t19\t39\tC3\r\n      3382  1FFFFFFF   00000004    8        00\t00\tFF\tFF\tFF\tFF\tFF\tFF\r\n      3423  0CF102A7   00000004    8        30\t75\tE0\t2E\t80\tFF\tFF\tFD\r\n      3423  0CF101A7   00000004    8        68\t00\t97\tCC\t00\t19\t39\tC5\r\n      3422  1FFFFFFF   00000004    8        00\t00\tFF\tFF\tFF\tFF\tFF\tFF\r\n      3412  1FFFFFFF   00000004    8        00\t00\tFF\tFF\tFF\tFF\tFF\tFF\r\n      3403  0CF102A7   00000004    8        30\t75\tE0\t2E\t80\tFF\tFF\tFD\r\n      3403  0CF101A7   00000004    8        68\t00\t97\tCC\t00\t19\t39\tC4\r\n      3402  1FFFFFFF   00000004    8        00\t00\tFF\tFF\tFF\tFF\tFF\tFF\r\n      3393  18F106A7   00000004    8        00\tF7\tFF\tFF\tFF\tFF\tFF\tB4\r\n      3392  1FFFFFFF   00000004    8        00\t00\tFF\tFF\tFF\tFF\tFF\tFF\r\n      3383  0CF102A7   00000004    8        30\t75\tE0\t2E\t80\tFF\tFF\tFD\r\n      3383  0CF101A7   00000004    8        68\t00\t97\tCC\t00\t19\t39\tC3\r\n      3432  1FFFFFFF   00000004    8        00\t00\tFF\tFF\tFF\tFF\tFF\tFF\r\n      3423  0CF102A7   00000004    8        30\t75\tE0\t2E\t80\tFF\tFF\tFD\r\n      3423  0CF101A7   00000004    8        68\t00\t97\tCC\t00\t19\t39\tC5\r\n      3422  1FFFFFFF   00000004    8        00\t00\tFF\tFF\tFF\tFF\tFF\tFF\r\n      3412  1FFFFFFF   00000004    8        00\t00\tFF\tFF\tFF\tFF\tFF\tFF\r\n      3403  0CF102A7   00000004    8        30\t75\tE0\t2E\t80\tFF\tFF\tFD\r\n      3403  0CF101A7   00000004    8        68\t00\t97\tCC\t00\t19\t39\tC4\r\n      3402  1FFFFFFF   00000004    8        00\t00\tFF\tFF\tFF\tFF\tFF\tFF\r\n      3393  18F106A7   00000004    8        00\tF7\tFF\tFF\tFF\tFF\tFF\tB4\r\n      3392  1FFFFFFF   00000004    8        00\t00\tFF\tFF\tFF\tFF\tFF\tFF\r\n      3383  0CF102A7   00000004    8        30\t75\tE0\t2E\t80\tFF\tFF\tFD\r\n      3441  18F11FF0   00000004    8        FF\t3F\t90\t68\t88\t1B\t10\tAC\r\n      3432  1FFFFFFF   00000004    8        00\t00\tFF\tFF\tFF\tFF\tFF\tFF\r\n      3423  0CF102A7   00000004    8        30\t75\tE0\t2E\t80\tFF\tFF\tFD\r\n      3423  0CF101A7   00000004    8        68\t00\t97\tCC\t00\t19\t39\tC5\r\n      3422  1FFFFFFF   00000004    8        00\t00\tFF\tFF\tFF\tFF\tFF\tFF\r\n      3412  1FFFFFFF   00000004    8        00\t00\tFF\tFF\tFF\tFF\tFF\tFF\r\n      3403  0CF102A7   00000004    8        30\t75\tE0\t2E\t80\tFF\tFF\tFD\r\n      3403  0CF101A7   00000004    8        68\t00\t97\tCC\t00\t19\t39\tC4\r\n      3402  1FFFFFFF   00000004    8        00\t00\tFF\tFF\tFF\tFF\tFF\tFF\r\n      3393  18F106A7   00000004    8        00\tF7\tFF\tFF\tFF\tFF\tFF\tB4\r\n      3392  1FFFFFFF   00000004    8        00\t00\tFF\tFF\tFF\tFF\tFF\tFF\r\n      3442  18F120F0   00000004    8        2B\t75\t60\tB1\tB0\t01\tFF\tFF\r\n      3441  18F11FF0   00000004    8        FF\t3F\t90\t68\t88\t1B\t10\tAC\r\n      3432  1FFFFFFF   00000004    8        00\t00\tFF\tFF\tFF\tFF\tFF\tFF\r\n      3423  0CF102A7   00000004    8        30\t75\tE0\t2E\t80\tFF\tFF\tFD\r\n      3423  0CF101A7   00000004    8        68\t00\t97\tCC\t00\t19\t39\tC5\r\n      3422  1FFFFFFF   00000004    8        00\t00\tFF\tFF\tFF\tFF\tFF\tFF\r\n      3412  1FFFFFFF   00000004    8        00\t00\tFF\tFF\tFF\tFF\tFF\tFF\r\n      3403  0CF102A7   00000004    8        30\t75\tE0\t2E\t80\tFF\tFF\tFD\r\n      3403  0CF101A7   00000004    8        68\t00\t97\tCC\t00\t19\t39\tC4\r\n      3402  1FFFFFFF   00000004    8        00\t00\tFF\tFF\tFF\tFF\tFF\tFF\r\n      3393  18F106A7   00000004    8        00\tF7\tFF\tFF\tFF\tFF\tFF\tB4\r\n      3443  0CF101A7   00000004    8        68\t00\t97\tCC\t00\t19\t39\tC6\r\n      3442  18F120F0   00000004    8        2B\t75\t60\tB1\tB0\t01\tFF\tFF\r\n      3441  18F11FF0   00000004    8        FF\t3F\t90\t68\t88\t1B\t10\tAC\r\n      3432  1FFFFFFF   00000004    8        00\t00\tFF\tFF\tFF\tFF\tFF\tFF\r\n      3423  0CF102A7   00000004    8        30\t75\tE0\t2E\t80\tFF\tFF\tFD\r\n      3423  0CF101A7   00000004    8        68\t00\t97\tCC\t00\t19\t39\tC5\r\n      3422  1FFFFFFF   00000004    8        00\t00\tFF\tFF\tFF\tFF\tFF\tFF\r\n      3412  1FFFFFFF   00000004    8        00\t00\tFF\tFF\tFF\tFF\tFF\tFF\r\n      3403  0CF102A7   00000004    8        30\t75\tE0\t2E\t80\tFF\tFF\tFD\r\n      3403  0CF101A7   00000004    8        68\t00\t97\tCC\t00\t19\t39\tC4\r\n      3402  1FFFFFFF   00000004    8        00\t00\tFF\tFF\tFF\tFF\tFF\tFF\r\n      3443  0C3C4D4A   00000004    8        BE\tFF\tFF\t7F\t18\tFF\tFF\t5A\r\n      3443  0CF101A7   00000004    8        68\t00\t97\tCC\t00\t19\t39\tC6\r\n      3442  18F120F0   00000004    8        2B\t75\t60\tB1\tB0\t01\tFF\tFF\r\n      3441  18F11FF0   00000004    8        FF\t3F\t90\t68\t88\t1B\t10\tAC\r\n      3432  1FFFFFFF   00000004    8        00\t00\tFF\tFF\tFF\tFF\tFF\tFF\r\n      3423  0CF102A7   00000004    8        30\t75\tE0\t2E\t80\tFF\tFF\tFD\r\n      3423  0CF101A7   00000004    8        68\t00\t97\tCC\t00\t19\t39\tC5\r\n      3422  1FFFFFFF   00000004    8        00\t00\tFF\tFF\tFF\tFF\tFF\tFF\r\n      3412  1FFFFFFF   00000004    8        00\t00\tFF\tFF\tFF\tFF\tFF\tFF\r\n      3403  0CF102A7   00000004    8        30\t75\tE0\t2E\t80\tFF\tFF\tFD\r\n      3403  0CF101A7   00000004    8        68\t00\t97\tCC\t00\t19\t39\t
